vi "get_bool_node_term.vi"(0 "Terms[] In":refnum<vi>[](array[refnum]), 11 "error in (no error)":errorcluster) -> (4 "Terms[]  Out":refnum<vi>[](array[refnum]), 6 "Pick Term":refnum<vi>, 8 "Enable Term":refnum<vi>, 10 "Disable Term":refnum<vi>, 14 "Output Term":refnum<vi>, 15 "error out":errorcluster)   [LabVIEW 2018]
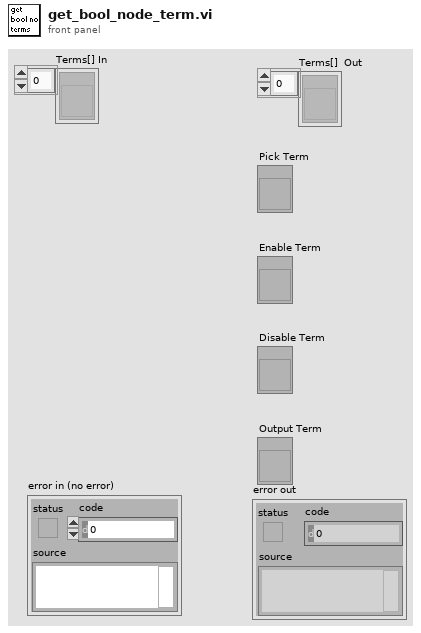
[diagram p1: front panel]
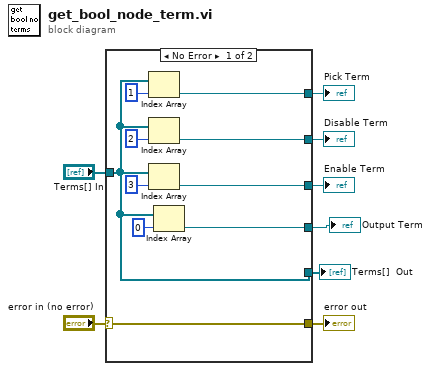
[diagram p0: block diagram]
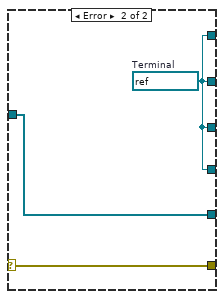
[diagram p2: hidden frame]
diagram:
  n1 = case shown="No Error" "error in (no error)" {
    selector: "error in (no error)" -> [w12 w21]
    tunnel: [w13 w19] -> w8
    tunnel: "Terms[] In" -> [w11 w20]
    tunnel: [w14 w19] -> w6
    tunnel: [w15 w19] -> w5
    tunnel: [w12 w21] -> w3
    tunnel: [w11 w20] -> w2
    tunnel: [w9 w19] -> w1
    frame No Error {
      n2 = Index Array(array=w11, index=1) -> (element=w13:refnum<vi>)
      n3 = Index Array(array=w11, index=2) -> (element=w14:refnum<vi>)
      n4 = Index Array(array=w11, index=3) -> (element=w15:refnum<vi>)
      n5 = Index Array(array=w11, index=0) -> (element=w9:refnum<vi>)
    }
    frame Error {
      w19 = refnum<vi> refnum  # Terminal
    }
  }
  "Pick Term" <- w8
  "Disable Term" <- w6
  "Enable Term" <- w5
  "error out" <- w3
  "Terms[]  Out" <- w2
  "Output Term" <- w1
